vi "Hill Expansion.vi"(7 "Robot Radius":u16, 10 "Boolean array":bool[](array[boolean]), 11 "RAW SICK Data":T1) -> (1 "Expansion Array":u16[](array[numeric]), 2 "Expanded Boolean Array":bool[](array[boolean]))   [LabVIEW 2009]
uses:
  TypeDefs/Sensor Typedefs/SICK Array.ctl
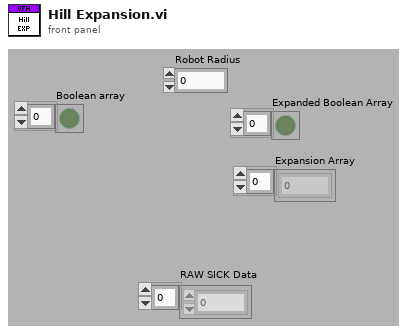
[diagram p1: front panel]
types:
  T1 = typedef "SICK Array.ctl" = u16[]
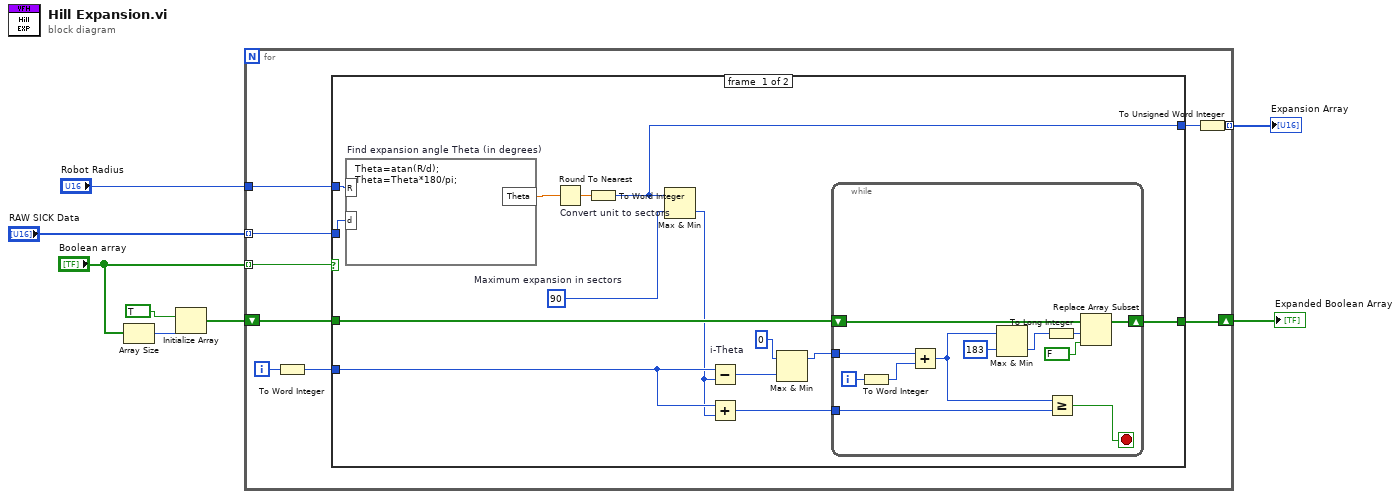
[diagram p0: block diagram]
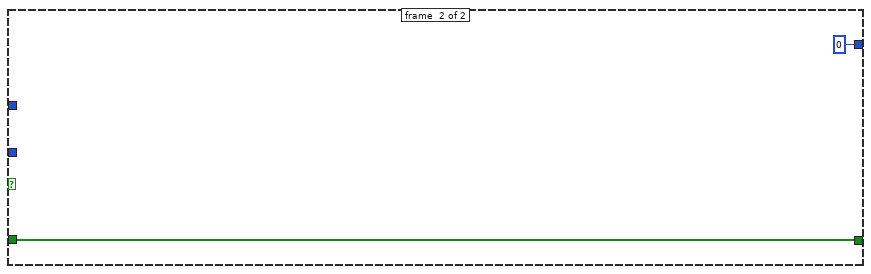
[diagram p2: hidden frame]
diagram:
  n1 = Array Size(array="Boolean array") -> (size(s)=w6:i32)
  n2 = Initialize Array(TRUE, w6) -> (w4:bool[])
  n3 = for {
    tunnel: "Boolean array" -> [w10] mode=indexing
    tunnel: "RAW SICK Data" -> [w17] mode=indexing
    tunnel: "Robot Radius" -> [w16]
    shift-right: [w12] -> w3
    shift-left: w4 -> [w15]
    tunnel: [w9] -> w2 mode=indexing
    i -> [w14]
    n4 = To Word Integer(number=w14) -> (16bit integer=w13:i16)
    n5 = case shown="False" w10 {
      tunnel: w17 -> [w31 _]
      tunnel: w16 -> [w30 _]
      tunnel: w15 -> [w29 w44]
      tunnel: w13 -> [w28 _]
      tunnel: [w27 w44] -> w12
      tunnel: [w26 i16 0] -> w11
      frame #0 {
        w18 = i16 90  # Maximum expansion in sectors
        n6 = formula code="Theta=atan(R/d);\nTheta=Theta*180/pi;" "Find expansion angle Theta (in degrees)"("R"=w30, "d"=w31) -> ("Theta"=w25:dbl)
        n7 = Round To Nearest "Convert unit to sectors"(number=w25) -> (nearest integer value=w24:dbl)
        n8 = To Word Integer(number=w24) -> (16bit integer=w26:i16)
        n9 = Max & Min(x=w26, y=w18) -> (min(x,y)=w19:i16)  [unwired: 1 out]
        n10 = Subtract "i-Theta"(x=w28, y=w19) -> (x-y=w23:i16)
        n11 = Add(x=w28, y=w19) -> (x+y=w22:i16)
        n12 = Max & Min(x=i16 0, y=w23) -> (max(x,y)=w20:i16)  [unwired: 1 out]
        n13 = while {
          shift-right: [w42] -> w27
          shift-left: w29 -> [w40]
          tunnel: w20 -> [w39]
          tunnel: w22 -> [w35]
          i -> [w38]
          stop <- w34 stop-if-true
          n14 = To Word Integer(number=w38) -> (16bit integer=w37:i16)
          n15 = Add(x=w39, y=w37) -> (x+y=w36:i16)
          n16 = Max & Min(x=w36, y=i16 183) -> (min(x,y)=w32:i16)  [unwired: 1 out]
          n17 = To Long Integer(number=w32) -> (32bit integer=w43:i32)
          n18 = Greater Or Equal?(x=w36, y=w35) -> (x >= y?=w34:bool)
          n19 = Replace Array Subset(array=w40, new element=FALSE, index=w43) -> (w42:bool[])
        }
      }
      frame #1 {
      }
    }
    n20 = To Unsigned Word Integer(number=w11) -> (unsigned 16bit integer=w9:u16)
  }
  "Expanded Boolean Array" <- w3
  "Expansion Array" <- w2
